vi "Run_3_of_5_Tests.vi"() -> ()   [LabVIEW 2019]
panel:
  out "Profiled PID Input/Output":bool
  out "State Space Util":bool
  out "Runge Kutta Time Varying":bool
  out "Swerve Drive Kinematics":bool
  out "Swerve Drive Odometry":bool
  out "All Tests Finished":bool
  out "Trajectory Concatenate":bool
  out "Timer":bool
  out "Single Jointed Arm Sim":bool
  out "Simple Motor Feedforward":bool
  out "Swerve Drive Pose Est":bool
  out "Swerve Module State":bool
  out "Slew Rate Limiter":bool
  out "Quintic Spline":bool
  out "Ramsete":bool
  out "Profiled PID":bool
  out "Rotation":bool
  out "Pose":bool
  out "PID tolerance":bool
  # "FORMAL TRAJECTORY / CONTROL LIBRARY TEST PROCEDURE"
  # "FUNCTION NOT\nIMPLEMENTED"
  # "Rectangular region constraint"
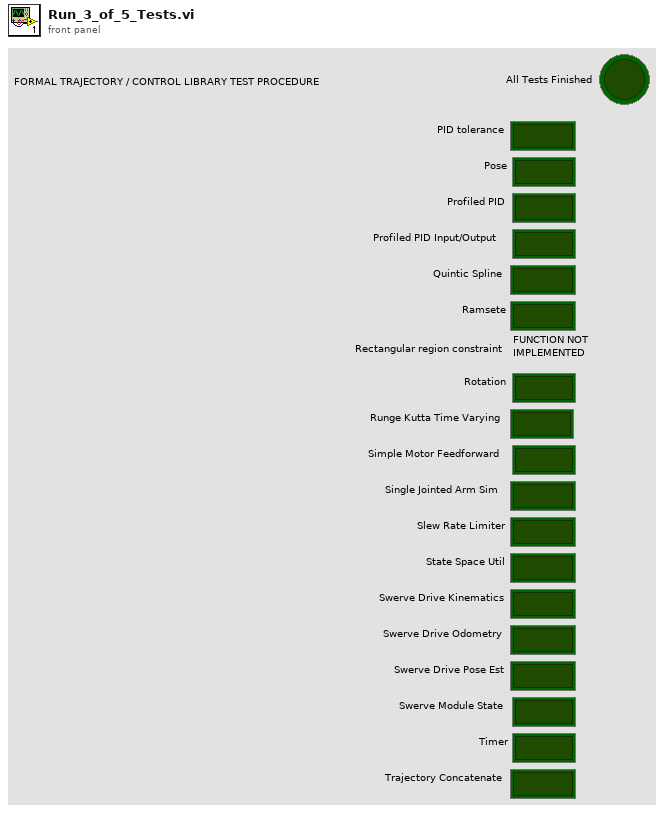
[diagram p1: front panel]
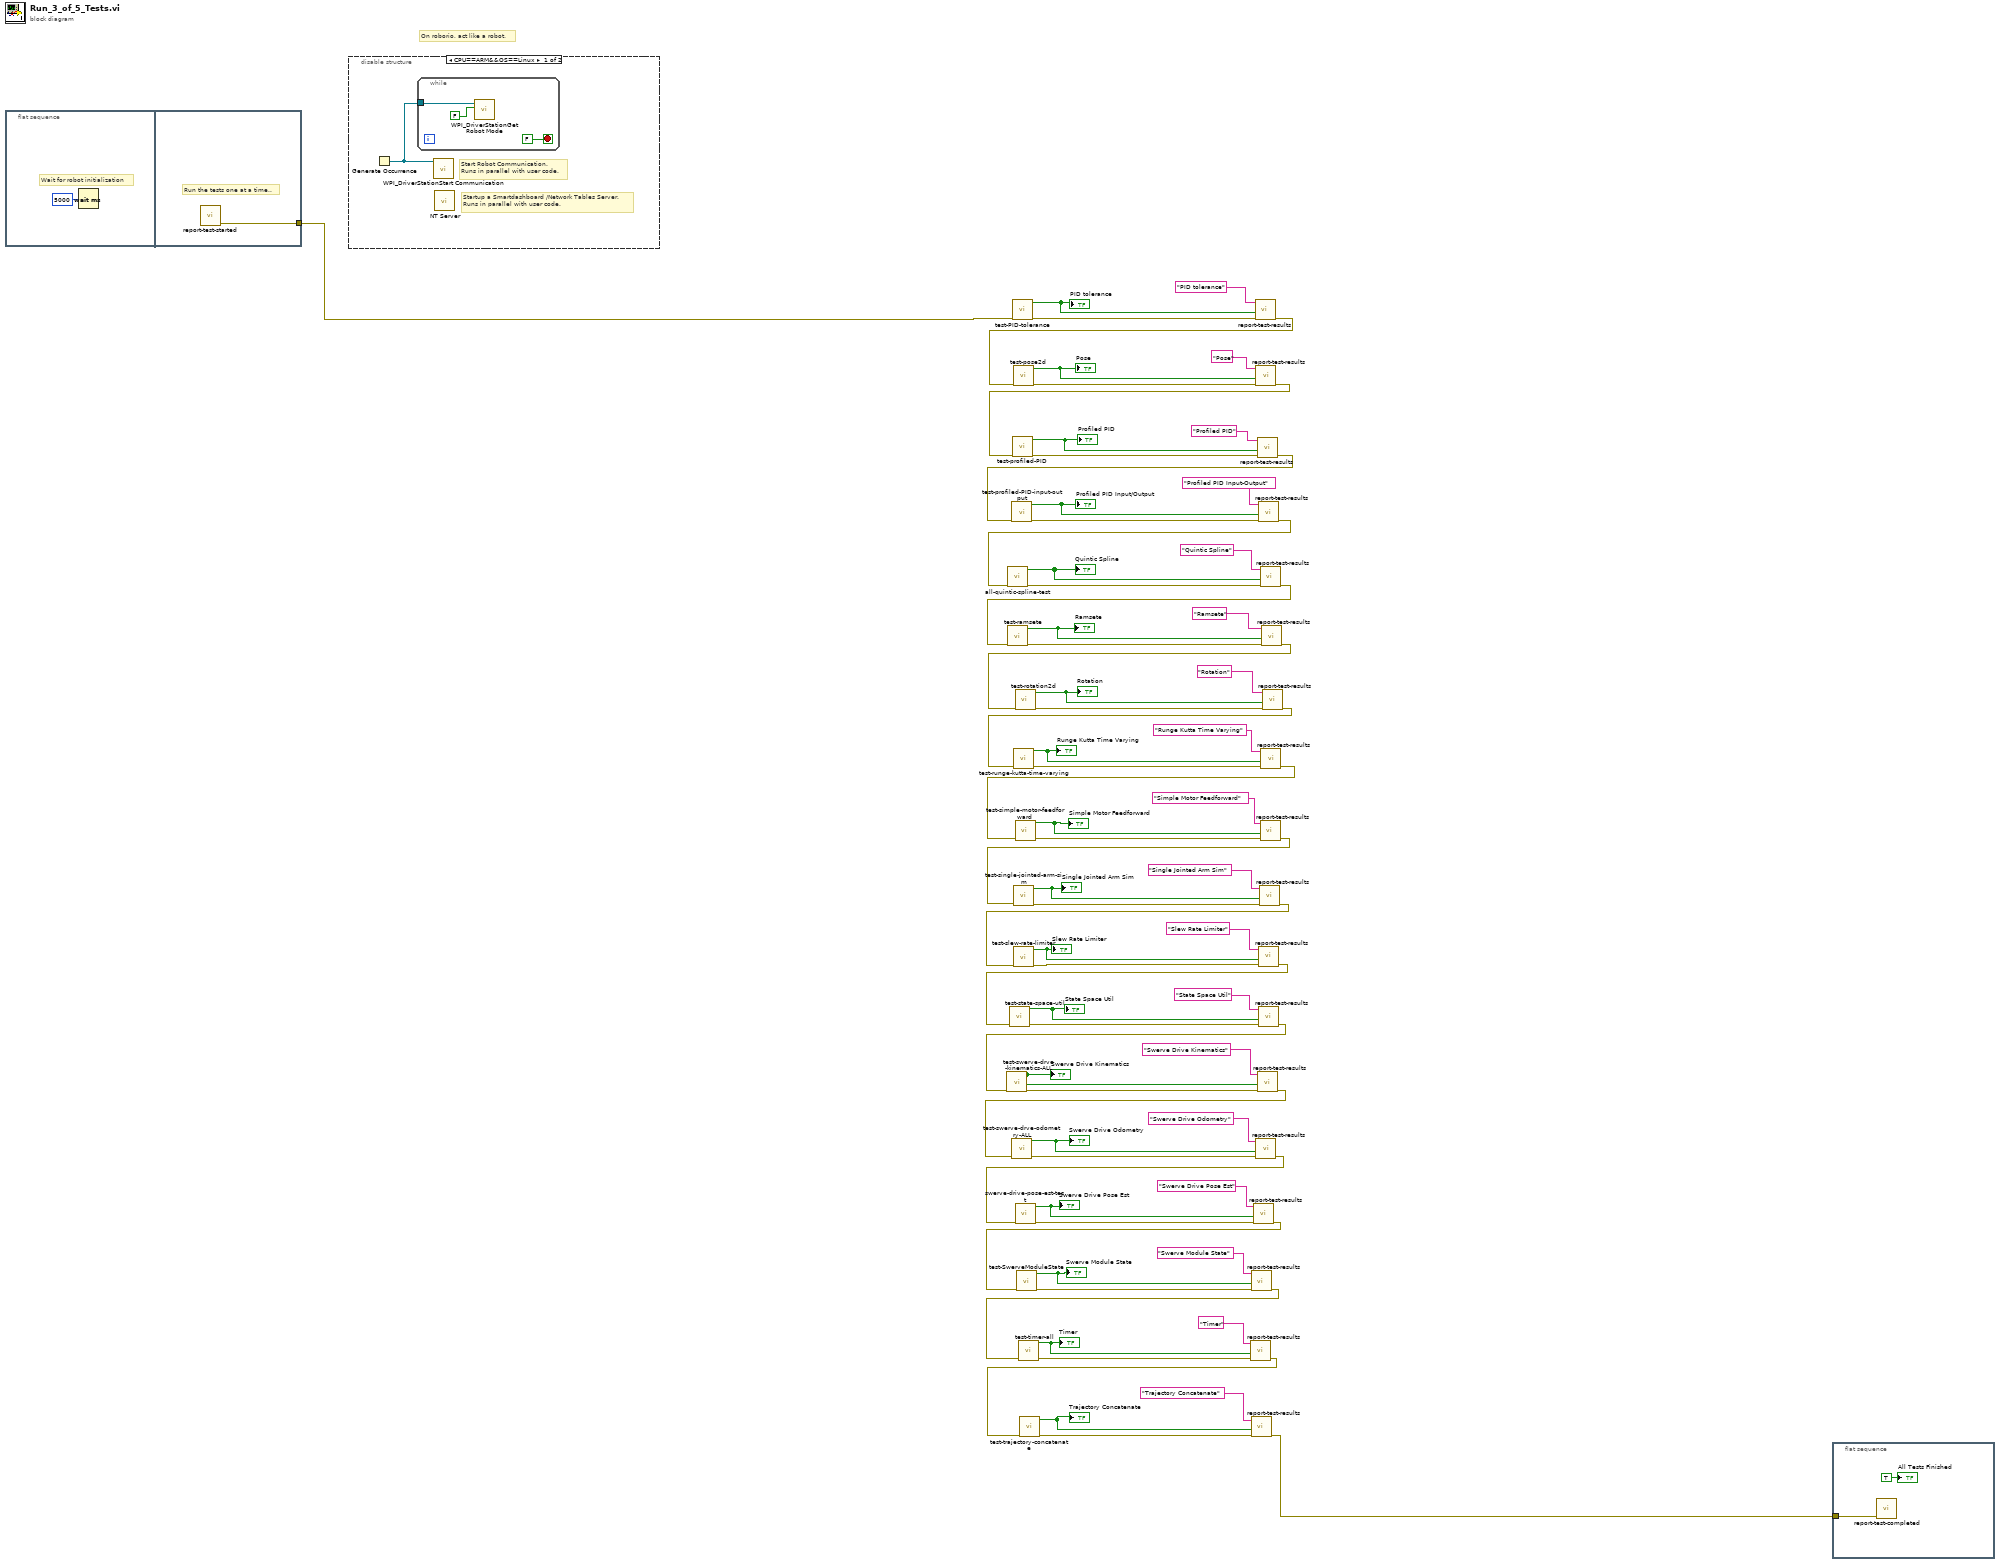
[diagram p0: block diagram]
diagram:
  # "On roborio, act like a robot."
  n1 = flat-sequence {
    tunnel: [w75] -> w1
    frame #0 {
      # "Wait for robot initialization"
      n2 = Wait (ms)(milliseconds to wait=u32 5000) -> ()  [unwired: 1 out]
    }
    frame #1 {
      # "Run the tests one at a time.."
      n3 = call "report-test-started.vi"() -> ("error out"=w75:errorcluster)  [unwired: 11 in]
    }
  }
  n4 = disable-structure shown="CPU==ARM&&OS==Linux" {
    frame condition #0 (active) {
      # "Startup a Smartdashboard /Network Tables Server.\nRuns in parallel with user code."
      # "Start Robot Communication.\nRuns in parallel with user code."
      n5 = Generate Occurrence() -> (w76:refnum<k4>)
      n6 = while {
        tunnel: w76 -> [w79]
        stop <- FALSE stop-if-true
        n7 = call <vilib>:"WPI_DriverStationGet Robot Mode.vi"("Finish"=FALSE, "DS Occurrence"=w79) -> ()  [unwired: 10 out]
      }
      n8 = call <vilib>:"WPI_DriverStationStart Communication.vi"("occurrence"=w76) -> ()  [unwired: 2 in, 9 out]
      n9 = call <vilib>:"NT Server.vi"() -> ()  [unwired: 12 in]
    }
    frame condition #1 {
    }
  }
  n10 = call "test-PID-tolerance.vi"("error in (no error)"=w1) -> ("error out"=w37:errorcluster, "All Tests Passed"=w70:bool)  [unwired: 9 in]
  "PID tolerance" <- w70
  n11 = call "report-test-results.vi"("error in (no error)"=w37, "TestPassed"=w70, "Test Name"="PID tolerance") -> ("error out"=w19:errorcluster)  [unwired: 8 in]
  n12 = call "test-pose2d.vi"("error in (no error)"=w19) -> ("error out"=w36:errorcluster, "All PASSED"=w71:bool)  [unwired: 9 in]
  "Pose" <- w71
  n13 = call "report-test-results.vi"("error in (no error)"=w36, "TestPassed"=w71, "Test Name"="Pose") -> ("error out"=w34:errorcluster)  [unwired: 8 in]
  n14 = call "test-profiled-PID.vi"("error in (no error)"=w34) -> ("error out"=w35:errorcluster, "Test Passed 0"=w58:bool)  [unwired: 9 in]
  "Profiled PID" <- w58
  n15 = call "report-test-results.vi"("error in (no error)"=w35, "TestPassed"=w58, "Test Name"="Profiled PID") -> ("error out"=w18:errorcluster)  [unwired: 8 in]
  n16 = call "test-profiled-PID-input-output.vi"("error in (no error)"=w18) -> ("error out"=w33:errorcluster, "All Tests Passed"=w57:bool)  [unwired: 9 in]
  "Profiled PID Input/Output" <- w57
  n17 = call "report-test-results.vi"("error in (no error)"=w33, "TestPassed"=w57, "Test Name"="Profiled PID Input-Output") -> ("error out"=w17:errorcluster)  [unwired: 8 in]
  n18 = call "all-quintic-spline-test.vi"("error in (no error)"=w17) -> ("error out"=w32:errorcluster, "ALL TESTS PASSED"=w56:bool)  [unwired: 9 in]
  "Quintic Spline" <- w56
  n19 = call "report-test-results.vi"("error in (no error)"=w32, "TestPassed"=w56, "Test Name"="Quintic Spline") -> ("error out"=w16:errorcluster)  [unwired: 8 in]
  n20 = call "test-ramsete.vi"("error in (no error)"=w16) -> ("error out"=w20:errorcluster, "AtReference End"=w55:bool)  [unwired: 9 in]
  "Ramsete" <- w55
  n21 = call "report-test-results.vi"("error in (no error)"=w20, "TestPassed"=w55, "Test Name"="Ramsete") -> ("error out"=w15:errorcluster)  [unwired: 8 in]
  n22 = call "test-rotation2d.vi"("error in (no error)"=w15) -> ("error out"=w21:errorcluster, "ALL TESTS PASSED"=w54:bool)  [unwired: 9 in]
  "Rotation" <- w54
  n23 = call "report-test-results.vi"("error in (no error)"=w21, "TestPassed"=w54, "Test Name"="Rotation") -> ("error out"=w14:errorcluster)  [unwired: 8 in]
  n24 = call "test-runge-kutta-time-varying.vi"("error in (no error)"=w14) -> ("error out"=w22:errorcluster, "Test Passed"=w53:bool)  [unwired: 9 in]
  "Runge Kutta Time Varying" <- w53
  n25 = call "report-test-results.vi"("error in (no error)"=w22, "TestPassed"=w53, "Test Name"="Runge Kutta Time Varying") -> ("error out"=w13:errorcluster)  [unwired: 8 in]
  n26 = call "test-simple-motor-feedforward.vi"("error in (no error)"=w13) -> ("error out"=w23:errorcluster, "All Tests Passed"=w52:bool)  [unwired: 9 in]
  "Simple Motor Feedforward" <- w52
  n27 = call "report-test-results.vi"("error in (no error)"=w23, "TestPassed"=w52, "Test Name"="Simple Motor Feedforward") -> ("error out"=w12:errorcluster)  [unwired: 8 in]
  n28 = call "test-single-jointed-arm-sim.vi"("error in (no error)"=w12) -> ("error out"=w24:errorcluster, "Test Passed"=w51:bool)  [unwired: 9 in]
  "Single Jointed Arm Sim" <- w51
  n29 = call "report-test-results.vi"("error in (no error)"=w24, "TestPassed"=w51, "Test Name"="Single Jointed Arm Sim") -> ("error out"=w11:errorcluster)  [unwired: 8 in]
  n30 = call "test-slew-rate-limiter.vi"("error in (no error)"=w11) -> ("error out"=w25:errorcluster, "All Tests Passed"=w50:bool)  [unwired: 9 in]
  "Slew Rate Limiter" <- w50
  n31 = call "report-test-results.vi"("error in (no error)"=w25, "TestPassed"=w50, "Test Name"="Slew Rate Limiter") -> ("error out"=w10:errorcluster)  [unwired: 8 in]
  n32 = call "test-state-space-util.vi"("error in (no error)"=w10) -> ("error out"=w26:errorcluster, "All Tests Passed"=w49:bool)  [unwired: 9 in]
  "State Space Util" <- w49
  n33 = call "report-test-results.vi"("error in (no error)"=w26, "TestPassed"=w49, "Test Name"="State Space Util") -> ("error out"=w9:errorcluster)  [unwired: 8 in]
  n34 = call "test-swerve-drve-kinematics-ALL.vi"("error in (no error)"=w9) -> ("error out"=w27:errorcluster, "ALL TEsts Passed"=w48:bool)  [unwired: 9 in]
  "Swerve Drive Kinematics" <- w48
  n35 = call "report-test-results.vi"("error in (no error)"=w27, "TestPassed"=w48, "Test Name"="Swerve Drive Kinematics") -> ("error out"=w8:errorcluster)  [unwired: 8 in]
  n36 = call "test-swerve-drve-odometry-ALL.vi"("error in (no error)"=w8) -> ("error out"=w28:errorcluster, "ALL TEsts Passed"=w45:bool)  [unwired: 9 in]
  "Swerve Drive Odometry" <- w45
  n37 = call "report-test-results.vi"("error in (no error)"=w28, "TestPassed"=w45, "Test Name"="Swerve Drive Odometry") -> ("error out"=w7:errorcluster)  [unwired: 8 in]
  n38 = call "swerve-drive-pose-est-test.vi"("error in (no error)"=w7) -> ("error out"=w29:errorcluster, "Test Passed"=w44:bool)  [unwired: 9 in]
  "Swerve Drive Pose Est" <- w44
  n39 = call "report-test-results.vi"("error in (no error)"=w29, "TestPassed"=w44, "Test Name"="Swerve Drive Pose Est") -> ("error out"=w6:errorcluster)  [unwired: 8 in]
  n40 = call "test-SwerveModuleState.vi"("error in (no error)"=w6) -> ("error out"=w30:errorcluster, "ALL TESTS PASSED"=w40:bool)  [unwired: 9 in]
  "Swerve Module State" <- w40
  n41 = call "report-test-results.vi"("error in (no error)"=w30, "TestPassed"=w40, "Test Name"="Swerve Module State") -> ("error out"=w5:errorcluster)  [unwired: 8 in]
  n42 = call "test-timer-all.vi"("error in (no error)"=w5) -> ("error out"=w4:errorcluster, "ALL TESTS PASSED"=w39:bool)  [unwired: 9 in]
  "Timer" <- w39
  n43 = call "report-test-results.vi"("error in (no error)"=w4, "TestPassed"=w39, "Test Name"="Timer") -> ("error out"=w3:errorcluster)  [unwired: 8 in]
  n44 = call "test-trajectory-concatenate.vi"("error in (no error)"=w3) -> ("error out"=w31:errorcluster, "TEsts Passed"=w38:bool)  [unwired: 9 in]
  "Trajectory Concatenate" <- w38
  n45 = call "report-test-results.vi"("error in (no error)"=w31, "TestPassed"=w38, "Test Name"="Trajectory Concatenate") -> ("error out"=w2:errorcluster)  [unwired: 8 in]
  n46 = flat-sequence {
    tunnel: w2 -> [w80]
    frame #0 {
      n47 = call "report-test-completed.vi"("error in (no error)"=w80) -> ()  [unwired: 10 in, 1 out]
      "All Tests Finished" <- TRUE ("All Tests Finished")
    }
  }
